vi "PR_Insert Production Record.vi"(7 "search_result":string="NG", 8 "error in (no error)":errorcluster, 9 "position":string="B", 10 "barcode":string="790", 11 "DBlink":string="Driver={ODBC Driver 17 for SQL Server};Server=localhost\\SQLEXPRESS;Database=ZDX201;UID=labview;PWD=Dsa@54137926") -> (0 "error out":errorcluster)   [LabVIEW 2019]
uses:
  <vilib>/addons/database/Connection.llb/DB Tools Open Connec (String).vi
  <vilib>/addons/database/NI_Database_API.lvlib
panel:
  in  "columns":string[](array[string])=["barcode", "position", "time_supply", "search_result", "workspace_id", "update_time"]
  in  "Insert value":T1={"barcode"="790", "position"="B", "Time_supply"=timestamp(3733883396.9235206 s since 1904-01-01), "search_result"="NG", "workspace_id"=1, "update_time"=timestamp(3733883396.9235206 s since 1904-01-01)} {"update_time" format="%<%.0X %x>T"; "Time_supply" format="%<%.0X %x>T"}
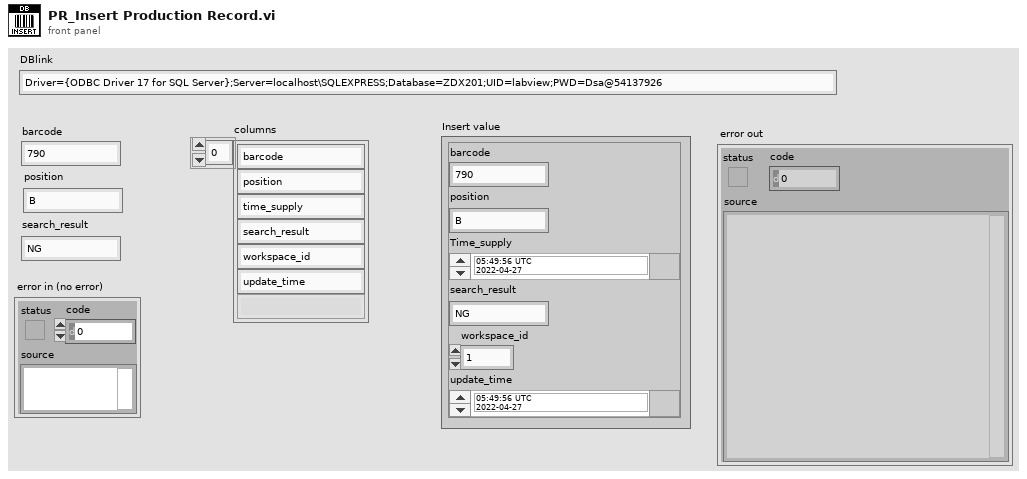
[diagram p1: front panel]
types:
  T1 = cluster{"barcode":string, "position":string, "Time_supply":timestamp, "search_result":string, "workspace_id":i16, "update_time":timestamp}
  T2 = typedef "NI_Database_API.lvlib/Conn ObjectReference.ctl" = refnum<k1>
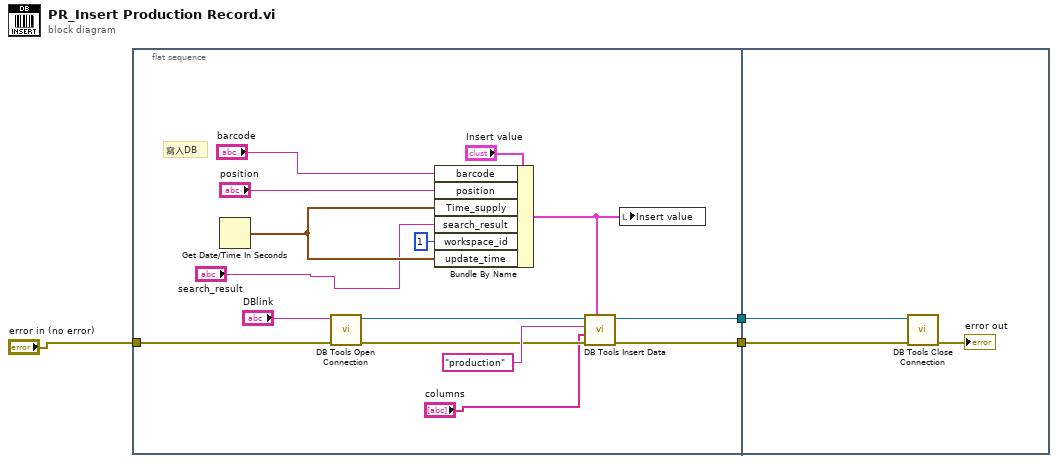
[diagram p0: block diagram]
diagram:
  n1 = flat-sequence {
    tunnel: [w17] -> w3
    tunnel: [w18] -> w2
    tunnel: "error in (no error)" -> [w5]
    tunnel: w3 -> [w19]
    tunnel: w2 -> [w20]
    frame #0 {
      # "寫入DB"
      n2 = Get Date/Time In Seconds() -> (seconds since 1Jan1904=w6:timestamp)
      n3 = call-poly <vilib>:"DB Tools Open Connection.vi"("error in (no error)"=w5, "connection information"="DBlink") -> ("error out"=w15:errorcluster, "connection reference"=w14:T2)  [unwired: 6 in]
      n4 = Bundle By Name(cluster="Insert value", "barcode"="barcode", "position"="position", "Time_supply"=w6, "search_result"="search_result", "workspace_id"=i16 1 ("workspace"), "update_time"=w6) -> (w11:T1)
      n5 = call <vilib>:"DB Tools Insert Data.vi"("data"=w11, "error in (no error)"=w15, "columns"="columns", "table"="production", "connection reference"=w14) -> ("error out"=w17:errorcluster, "connection reference out"=w18:T2)  [unwired: 5 in]
      n6 = local write "Insert value"(w11) -> ()
    }
    frame #1 {
      n7 = call <vilib>:"DB Tools Close Connection.vi"("error in (no error)"=w19, "connection reference"=w20) -> ("error out"=→"error out":errorcluster)  [unwired: 5 in]
    }
  }
